vi "Channel ID to Tree Items.vi"(8 "error in (no error)":errorcluster, 9 "Channel ID":string, 11 "Application Data in":T2) -> (0 "error out":errorcluster, 1 "Settings":T1, 2 "Item":T1, 3 "Application Data out":T2)   [LabVIEW 2017, in "DSF Data Viewer.lvlib"]
uses:
  DSF Data Viewer.lvlib
  Main VI/Application Data.ctl
  Builds/Data Sharing Framework/Current/Core/DSF Core.lvlibp/Engine/Classes/Framework/Framework.lvclass
  <vilib>/NI/Memory Manager/Classes/Pointer/Pointer.lvclass
  Buffer Reader/Buffer Data.ctl
  Builds/Data Sharing Framework/Current/Core/DSF Core.lvlibp/Engine/Classes/Buffer/Buffer.lvclass
  Tree Item.ctl
  Tree Item Type.ctl
  Builds/Data Sharing Framework/Current/Core/DSF Core.lvlibp/DSF Configuration API/Configuration Session.lvclass
  Builds/Data Sharing Framework/Current/Core/DSF Core.lvlibp/DSF Configuration API/Public/Read Item/Read Channel.vi
  Builds/Data Sharing Framework/Current/Core/DSF Core.lvlibp/DSF Configuration API/Public/Read Item/Read Settings.vi
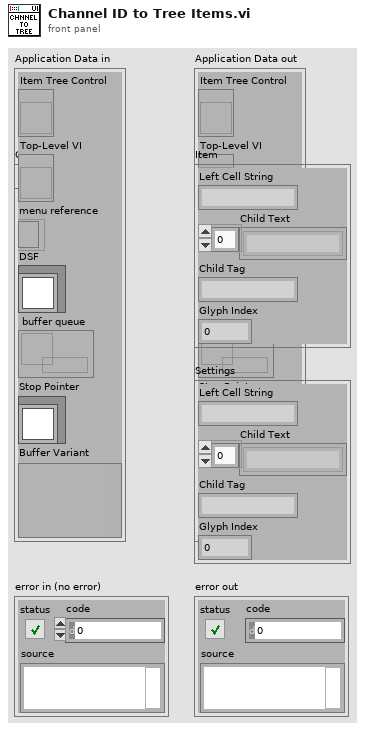
[diagram p1: front panel]
types:
  T1 = typedef "DSF Data Viewer.lvlib/Tree Item.ctl" = cluster{"Left Cell String":string, "Child Text":string[], "Child Tag":string, "Glyph Index":i32}
  T2 = typedef "DSF Data Viewer.lvlib/Application Data.ctl" = cluster{"Item Tree Control":refnum<vi>, "Top-Level VI":refnum<vi>, "menu reference":refnum<k9>, "DSF":refnum<class "Framework.lvclass">, "buffer queue":refnum<queue>, "Stop Pointer":refnum<class "Pointer.lvclass">, "Buffer Variant":variant}
  T3 = typedef "DSF Data Viewer.lvlib/Tree Item Type.ctl" = enum16{"Framework", "Plugin Group", "Plugin", "Group", "Transfer", "Buffer", "Channel"}
  T4 = typedef "DSF Core.lvlibp/DSF Channel Info.ctl" = cluster{"string buffer offset":u64, "string data type":T5, "engine data type":T5, "settings id":string}
  T5 = typedef "DSF Core.lvlibp/DSF Data Type.ctl" = enum8{"Bool", "SGL", "DBL", "I8", "I16", "I32", "I64", "U8", "U16", "U32", "U64"}
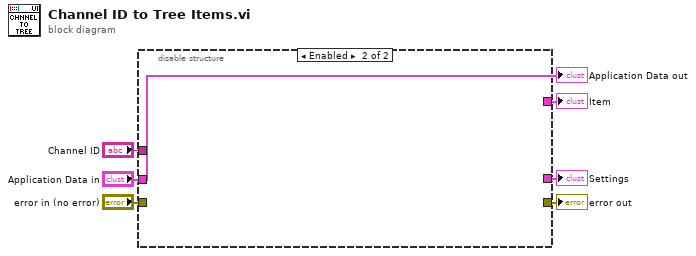
[diagram p0: block diagram]
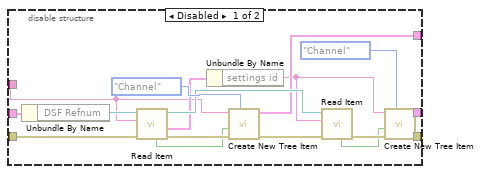
[diagram p2: hidden frame]
diagram:
  n1 = disable-structure shown="Enabled" {
    disable-tunnel: [w21 _] -> w6
    disable-tunnel: "error in (no error)" -> [w17 _]
    disable-tunnel: "Application Data in" -> [w13 _]
    disable-tunnel: [w12 _] -> w3
    disable-tunnel: [w11 _] -> w2
    disable-tunnel: "Channel ID" -> [w10 _]
    frame Disabled {
      n2 = Unbundle By Name(w13) -> ("DSF Refnum"=w14:refnum<class "Configuration Session.lvclass">)
      n3 = call-poly "Read Item.vi"("error in (no error)"=w17, "Channel ID"=w10, "Configuration Session in"=w14) -> ("error out"=w18:errorcluster, "value"=w15:T4, "Configuration Session out"=w16:refnum<class "Configuration Session.lvclass">, "found?"=w9:bool)  [unwired: 5 in]
      n4 = Unbundle By Name(w15) -> ("settings id"=w8:string)
      n5 = call "Create New Tree Item.vi"("Item Type"=Tree_Item_Type."Channel", "error in"=w18, "found?"=w9, "Left Cell String"=w10) -> ("error out"=w19:errorcluster, "Item"=w12:T1)  [unwired: 6 in]
      n6 = call-poly "Read Item.vi"("error in (no error)"=w19, "Settings ID"=w8, "Configuration Session in"=w16) -> ("error out"=w20:errorcluster, "found?"=w7:bool)  [unwired: 5 in, 2 out]
      n7 = call "Create New Tree Item.vi"("Item Type"=Tree_Item_Type."Channel", "error in"=w20, "found?"=w7, "Left Cell String"=w8) -> ("error out"=w21:errorcluster, "Item"=w11:T1)  [unwired: 6 in]
    }
    frame Enabled {
    }
  }
  "error out" <- w6
  "Item" <- w3
  "Settings" <- w2
  "Application Data out" <- "Application Data in"
